vi "Main RT.vi"() -> ()   [LabVIEW 2020]
uses:
  <vilib>/rvi/interface/nirviOpenFPGA/nirviOpenFPGA.xnode
  <vilib>/rvi/interface/nirviCloseFPGA/nirviCloseFPGA.xnode
  <vilib>/FPGAPlugInAG/Dynamic/niLvFpga_Close_Dynamic.vi
  <vilib>/rvi/interface/nirviReadWriteControl/nirviReadWriteControl.xnode
  NiFpgaLv.dll
  <vilib>/Utility/error.llb/Error Cluster From Error Code.vi
  <vilib>/rvi/interface/Simulation/niFpgaSimulationCallBeginRW.vi
  <vilib>/rvi/errors/niLvFpgaAdjustHostInterfaceError.vi
  Type Definitions/Acelerometer data--cluster.ctl
  Type Definitions/Shared.lvlib
  C:/Users/juan_/Desktop/Firebase Sesion 5 - FPGA/Type Definitions/Acelerometer data--cluster.ctl
  FPGA Bitfiles/firebasemyriofpg_FPGATarget_MainFPGA_NcPxUbWwTmc.lvbitx
  Firebase Sesion 5 - FPGA/FPGA/Main FPGA.vi
  <vilib>/FPGAPlugInAG/myRIO-1900/niLvFpga_Open_myRIO-1900.vi
  <vilib>/rvi/interface/common/dynamic/niFpgaDynamicAddResources.vi
panel:
  in  "stop":bool
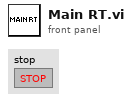
[diagram p1: front panel]
types:
  T1 = typedef "Shared.lvlib/Acelerometer data--cluster.ctl" = cluster{"X-Axis":dbl, "Y-Axis":dbl, "Z-Axis":dbl}
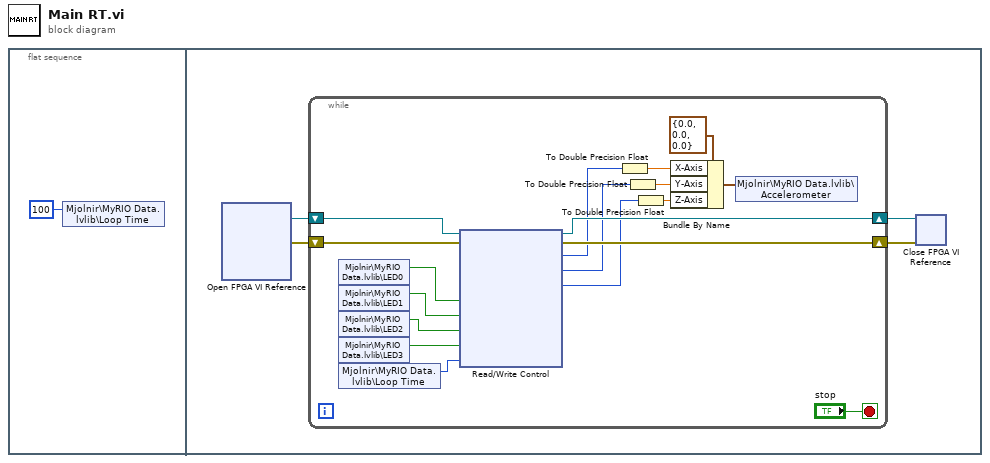
[diagram p0: block diagram]
diagram:
  n1 = flat-sequence {
    frame #0 {
      n2 = shared-variable "Mjolnir\\MyRIO Data.lvlib\\Loop Time"(u32 100 ("Loop Time")) -> ()  [unwired: 1 in, 1 out]
    }
    frame #1 {
      n3 = xnode "Open FPGA VI Reference"() -> ("FPGA VI Reference Out"=w3:refnum<k20>, "error out"=w5:errorcluster)  [unwired: 2 in]
      n4 = while {
        shift-right: [w22] -> w4
        shift-left: w5 -> [w23]
        shift-right: [w20] -> w2
        shift-left: w3 -> [w21]
        stop <- "stop" stop-if-true
        n5 = shared-variable "Mjolnir\\MyRIO Data.lvlib\\LED0"() -> (w10:bool)  [unwired: 1 in, 1 out]
        n6 = shared-variable "Mjolnir\\MyRIO Data.lvlib\\LED1"() -> (w9:bool)  [unwired: 1 in, 1 out]
        n7 = shared-variable "Mjolnir\\MyRIO Data.lvlib\\LED2"() -> (w8:bool)  [unwired: 1 in, 1 out]
        n8 = shared-variable "Mjolnir\\MyRIO Data.lvlib\\LED3"() -> (w7:bool)  [unwired: 1 in, 1 out]
        n9 = shared-variable "Mjolnir\\MyRIO Data.lvlib\\Loop Time"() -> (w6:u32)  [unwired: 1 in, 1 out]
        n10 = xnode "Read/Write Control"("FPGA VI Reference In"=w21, "error in"=w23, "LED0"=w10, "LED1"=w9, "LED2"=w8, "LED3"=w7, "Loop Time (ms)"=w6) -> ("FPGA VI Reference Out"=w20:refnum<k20>, "error out"=w22:errorcluster, "AccelerationX"=w16:i16, "AccelerationY"=w15:i16, "AccelerationZ"=w14:i16)
        n11 = To Double Precision Float(number=w16) -> (double precision float=w13:dbl)
        n12 = To Double Precision Float(number=w15) -> (double precision float=w12:dbl)
        n13 = To Double Precision Float(number=w14) -> (double precision float=w11:dbl)
        n14 = Bundle By Name(cluster=T1 {"X-Axis"=0.0, "Y-Axis"=0.0, "Z-Axis"=0.0} ("Acceleration"), "X-Axis"=w13, "Y-Axis"=w12, "Z-Axis"=w11) -> (w18:T1)
        n15 = shared-variable "Mjolnir\\MyRIO Data.lvlib\\Accelerometer"(w18) -> ()  [unwired: 1 in, 1 out]
      }
      n16 = xnode "Close FPGA VI Reference"("FPGA VI Reference In"=w2, "error in"=w4) -> ()  [unwired: 1 out]
    }
  }
